vi "IMAQ FPGA CXP EOI Generator.vi"(7 "Reset":bool, 9 "Height":u16, 10 "Enable":bool, 11 "EOL":bool) -> (3 "EOI":bool)   [LabVIEW 2020]
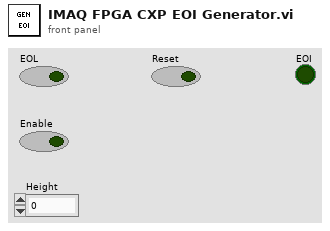
[diagram p1: front panel]
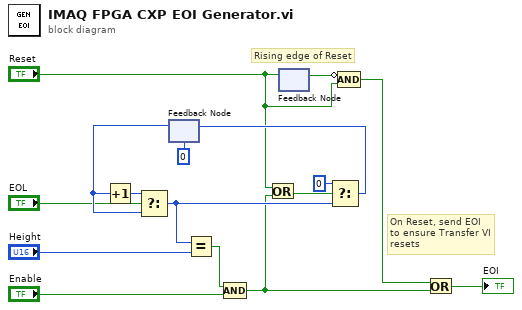
[diagram p0: block diagram]
diagram:
  # "On Reset, send EOI\nto ensure Transfer VI\nresets"
  # "Rising edge of Reset"
  n1 = feedback #1(u16 0) -> (w16:u16)
  n2 = Increment(x=w16) -> (x+1=w13:u16)
  n3 = Select(t=w13, s="EOL", f=w16) -> (s? t:f=w12:u16)
  n4 = Equal?(x=w12, y="Height") -> (x = y?=w11:bool)
  n5 = Compound Arithmetic op=AND(w11, "Enable") -> (w2:bool)
  n6 = Or(x="Reset", y=w2) -> (x .or. y?=w9:bool)
  n7 = feedback-in #2("Reset") -> ()
  n8 = feedback #2() -> (w5:bool)  [unwired: 1 in]
  n9 = Select(t=u16 0, s=w9, f=w12) -> (s? t:f=w14:u16)
  n10 = feedback-in #1(w14) -> ()
  n11 = Compound Arithmetic op=AND(invert w5, "Reset") -> (w3:bool)
  n12 = Or(x=w3, y=w2) -> (x .or. y?=→"EOI":bool)
